vi "Log_debug.vi"(9 "Total_samples":i32, 10 "File#":i32, 11 "Total_Records":i32) -> ()   [LabVIEW 2017]
panel:
  out "error out":errorcluster
  out "JSON string":string
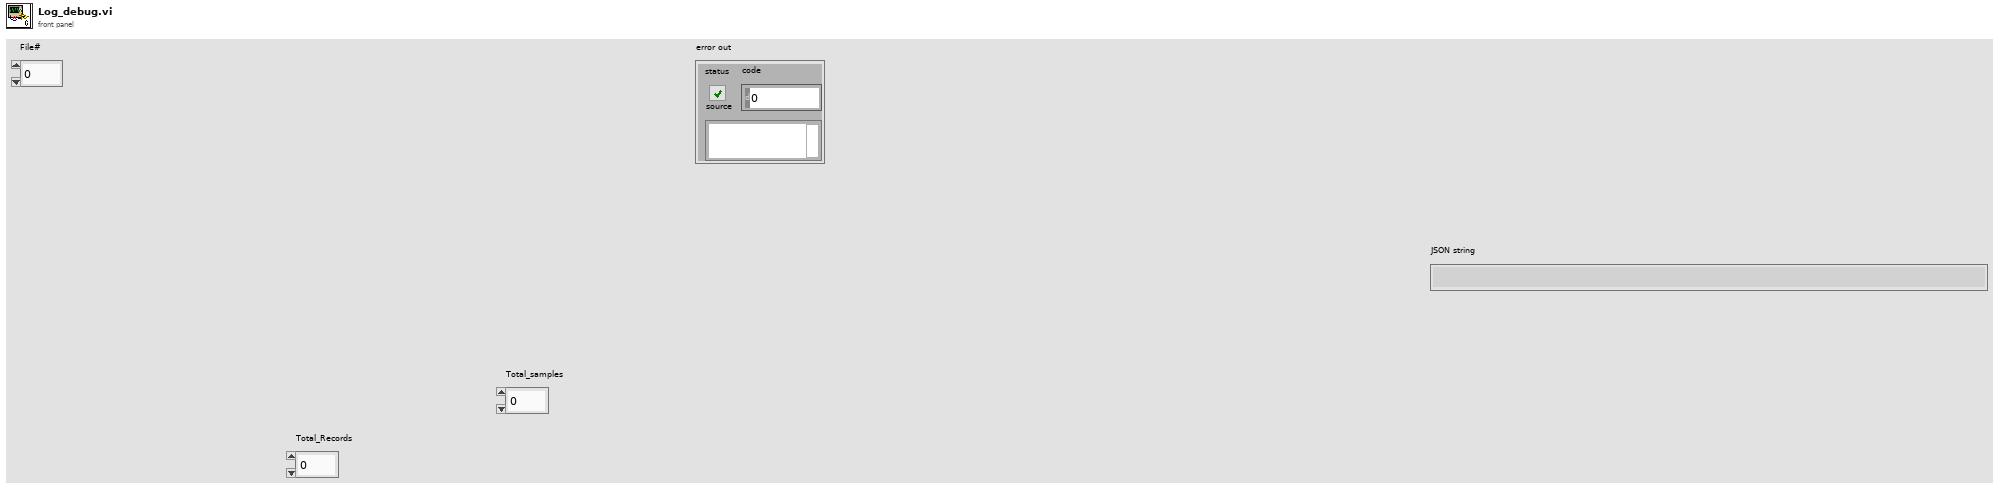
[diagram p1: front panel]
types:
  T1 = enum16{"open", "replace", "create", "open or create", "replace or create", "replace or create with confirmation"}
  T2 = cluster{"File#":i32, "Total_samples":i32, "Total_Records":i32}
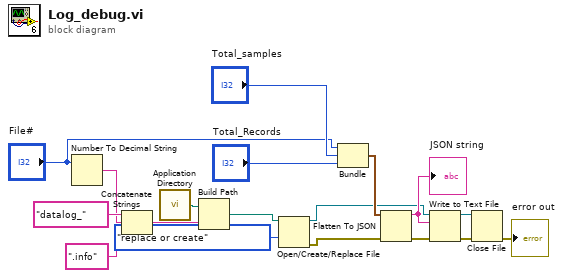
[diagram p0: block diagram]
diagram:
  n1 = Number To Decimal String(number="File#") -> (decimal integer string=w17:string)  [unwired: 1 in]
  n2 = Concatenate Strings("datalog_" ("string"), w17, ".info" ("string")) -> (w14:string)
  n3 = call <vilib>:"Application Directory.vi"() -> ("Application Directory"=w15:path)
  n4 = Build Path(base path=w15, name or relative path=w14) -> (appended path=w5:path)
  n5 = Open/Create/Replace File(file path (use dialog)=w5, operation (0:open)=T1."replace or create") -> (refnum out=w4:refnum<file>, error out=w2:errorcluster)  [unwired: 4 in, 1 out]
  n6 = Bundle("File#"="File#", "Total_samples"="Total_samples", "Total_Records"="Total_Records") -> (w7:T2)  [unwired: 1 in]
  n7 = Flatten To JSON(anything=w7, error in (no error)=w2) -> (JSON string=w10:string, 11:w11:errorcluster)  [unwired: 1 in]
  "JSON string" <- w10
  n8 = Write to Text File(file (use dialog)=w4, text=w10, error in=w11) -> (refnum out=w9:refnum<file>, error out=w8:errorcluster)  [unwired: 1 in, 1 out]
  n9 = Close File(refnum=w9, error in=w8) -> (error out=→"error out":errorcluster)  [unwired: 1 out]
